vi "calc_cap_ind.vi"(10 "R+jX":cluster{"R":dbl, "jX":dbl}, 11 "freq":dbl) -> (3 "R_Cap_Ind":T1)   [LabVIEW 2025]
panel:
  out "Cp":dbl
  out "Lp":dbl
  out "Xp":dbl
  out "Rp":dbl
  out "Z":dbl
  out "Cs":dbl
  out "Ls":dbl
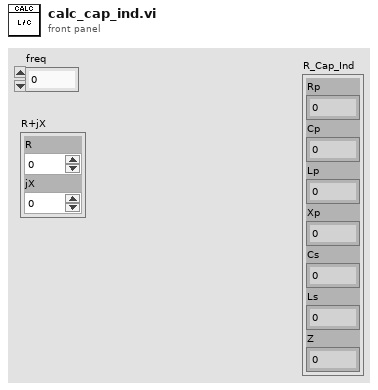
[diagram p1: front panel]
types:
  T1 = cluster{"Rp":dbl, "Cp":dbl, "Lp":dbl, "Xp":dbl, "Cs":dbl, "Ls":dbl, "Z":dbl}
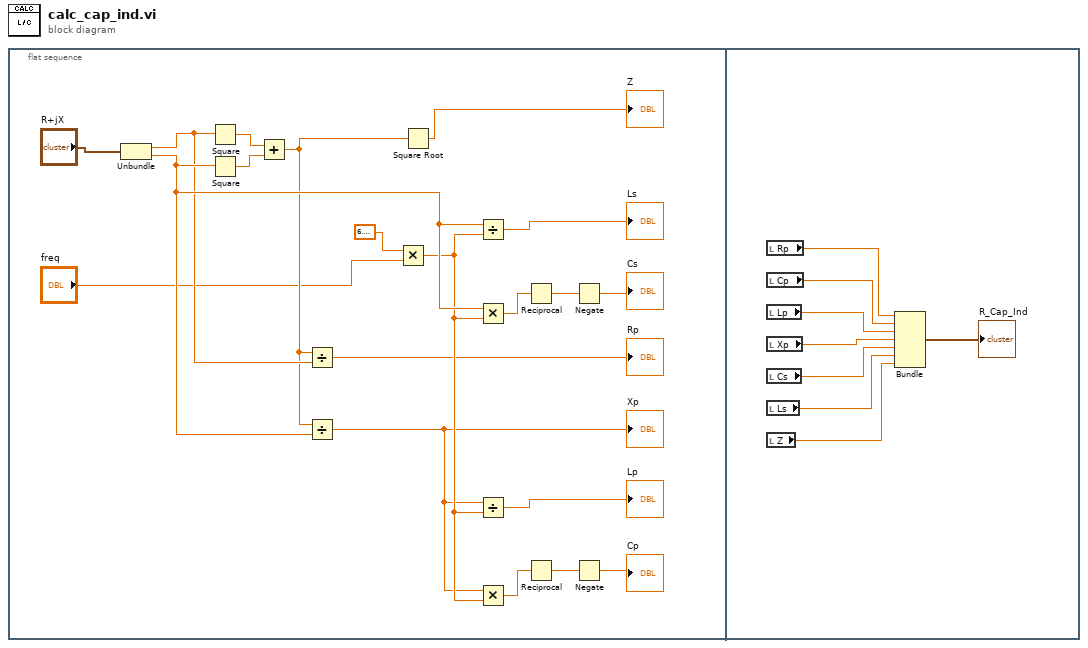
[diagram p0: block diagram]
diagram:
  n1 = flat-sequence {
    frame #0 {
      n2 = Unbundle("R+jX") -> ("R"=w19:dbl, "jX"=w20:dbl)
      n3 = Square(x=w19) -> (x^2=w4:dbl)
      n4 = Square(x=w20) -> (x^2=w5:dbl)
      n5 = Add(x=w4, y=w5) -> (x+y=w8:dbl)
      n6 = Divide(x=w8, y=w19) -> (x/y=→"Rp":dbl)
      n7 = Divide(x=w8, y=w20) -> (x/y=w12:dbl)
      "Xp" <- w12
      n8 = Multiply(x=6.283185307179586, y="freq") -> (x*y=w13:dbl)
      n9 = Square Root(x=w8) -> (sqrt(x)=→"Z":dbl)
      n10 = Divide(x=w20, y=w13) -> (x/y=→"Ls":dbl)
      n11 = Multiply(x=w20, y=w13) -> (x*y=w10:dbl)
      n12 = Divide(x=w12, y=w13) -> (x/y=→"Lp":dbl)
      n13 = Multiply(x=w12, y=w13) -> (x*y=w11:dbl)
      n14 = Reciprocal(x=w10) -> (1/x=w14:dbl)
      n15 = Reciprocal(x=w11) -> (1/x=w16:dbl)
      n16 = Negate(x=w14) -> (-x=→"Cs":dbl)
      n17 = Negate(x=w16) -> (-x=→"Cp":dbl)
    }
    frame #1 {
      n18 = local read "Rp"() -> (w21:dbl)
      n19 = local read "Cp"() -> (w22:dbl)
      n20 = local read "Lp"() -> (w23:dbl)
      n21 = local read "Xp"() -> (w24:dbl)
      n22 = local read "Cs"() -> (w25:dbl)
      n23 = local read "Ls"() -> (w26:dbl)
      n24 = local read "Z"() -> (w27:dbl)
      n25 = Bundle("Rp"=w21, "Cp"=w22, "Lp"=w23, "Xp"=w24, "Cs"=w25, "Ls"=w26, "Z"=w27) -> (→"R_Cap_Ind":T1)  [unwired: 1 in]
    }
  }
